vi "GetOpenDataEvents.vi"(8 "error in (no error)":errorcluster, 10 "data group":string, 11 "config":T1) -> (0 "error out":errorcluster, 2 "open data event configs":T2[](array[typedef]), 3 "open data events":T8[](array[typedef]))   [LabVIEW 2017, in "McsaDataEventCreator.lvlib"]
uses:
  <vilib>/addons/InsightCM/Devices/Shared/Mcsa/McsaDataEventCreator/McsaDataEventCreator.lvlib
  <vilib>/addons/InsightCM/Devices/Shared/Common/DataEvent/controls/Event.ctl
  <vilib>/addons/InsightCM/MessageBus/Base/controls/DataEvent.ctl
  <vilib>/addons/InsightCM/MessageBus/Base/controls/KeyValuePair.ctl
  <vilib>/addons/InsightCM/Devices/Shared/Common/DataEvent/controls/DataSet.ctl
  <vilib>/addons/InsightCM/MessageBus/Base/controls/DataSetMetadata.ctl
  <vilib>/addons/InsightCM/MessageBus/Base/controls/TrendPoint.ctl
  <vilib>/addons/InsightCM/MessageBus/Base/controls/TrendAlarmUpdate.ctl
  <vilib>/addons/InsightCM/MessageBus/Base/controls/TrendAlarmTransition.ctl
  <vilib>/addons/InsightCM/Devices/Shared/Mcsa/McsaDataEventCreator/controls/DataEventConfig.ctl
  <vilib>/addons/InsightCM/Devices/Shared/Mcsa/McsaDataEventCreator/controls/AcqParams.ctl
  <vilib>/addons/InsightCM/Devices/Shared/Common/DataAccumulator/controls/AccumulationSettings.ctl
  <vilib>/addons/InsightCM/Devices/Shared/Common/DataAccumulator/controls/accumulationType.ctl
  <vilib>/addons/InsightCM/Devices/Shared/Common/DVRBuffer/controls/BufferLocation.ctl
  <vilib>/addons/PointValueMap/controls/PointMap.ctl
  <vilib>/addons/InsightCM/Devices/Shared/Mcsa/McsaDataEventCreator/controls/config.ctl
  <vilib>/addons/PointValueMap/PointValueMap.lvlib
  <vilib>/addons/InsightCM/Devices/Shared/Common/DVRBuffer/DVRBuffer.lvlib
  <vilib>/addons/InsightCM/Devices/Shared/Common/DataAccumulator/DataAccumulator.lvlib
  <vilib>/addons/InsightCM/Devices/Shared/Common/DataEvent/DataEvent.lvlib
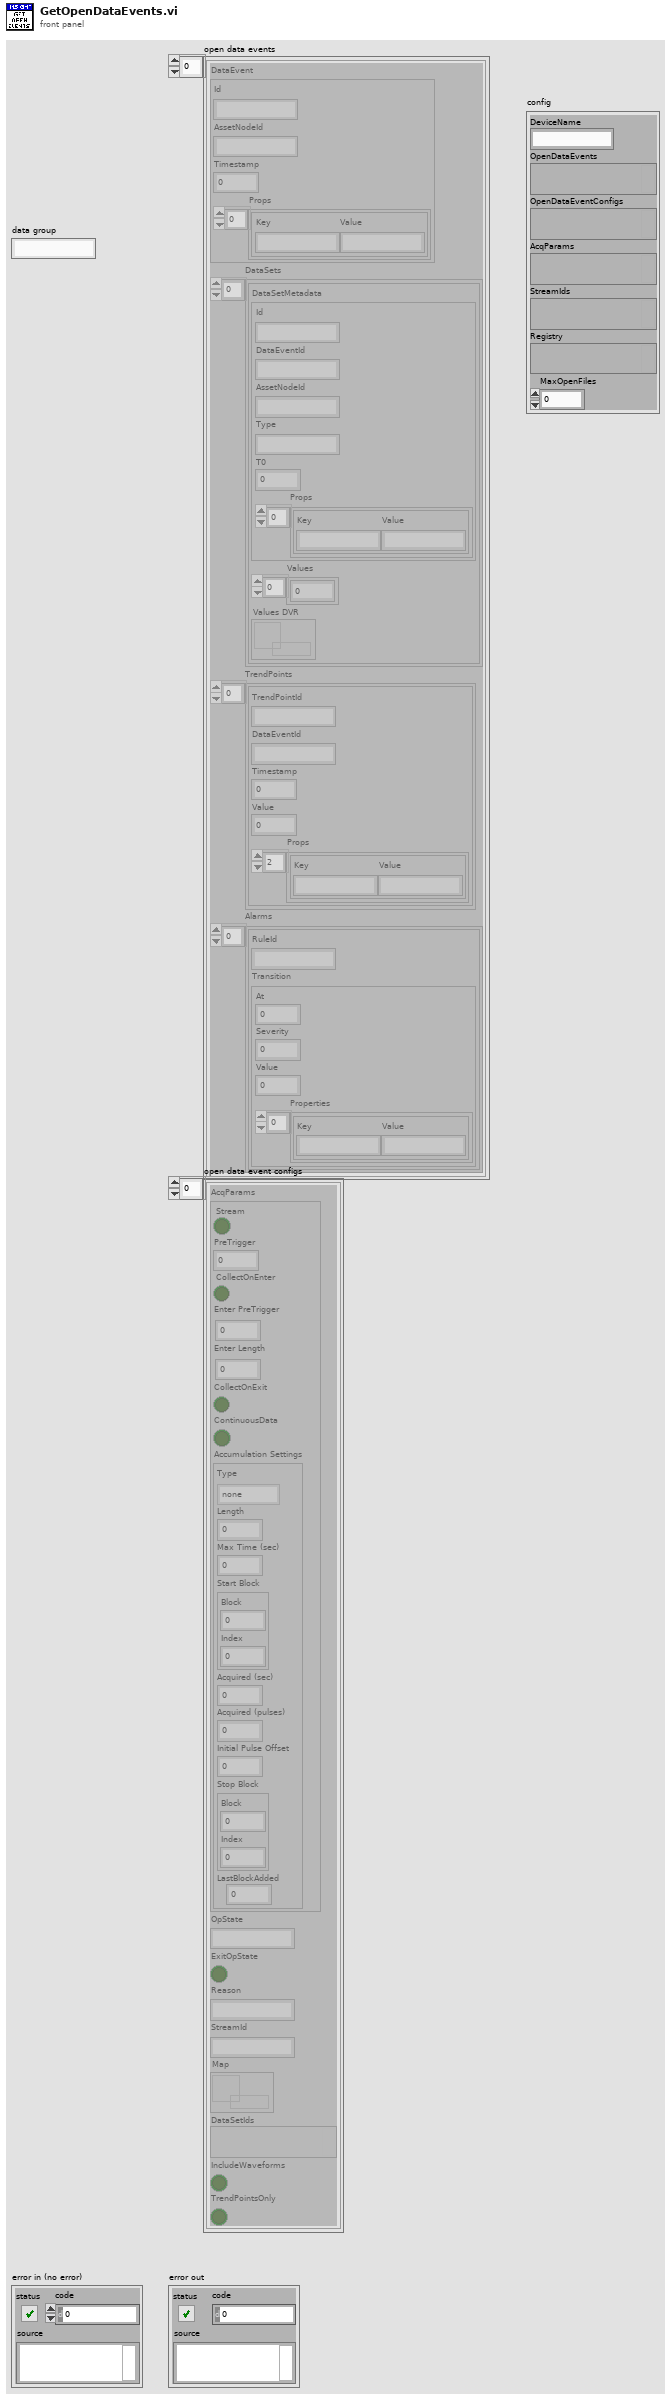
[diagram p1: front panel]
types:
  T1 = typedef "McsaDataEventCreator.lvlib/config.ctl" = cluster{"DeviceName":string, "OpenDataEvents":variant, "OpenDataEventConfigs":variant, "AcqParams":variant, "StreamIds":variant, "Registry":variant, "MaxOpenFiles":i32}
  T2 = typedef "McsaDataEventCreator.lvlib/DataEventConfig.ctl" = cluster{"AcqParams":T3, "OpState":string, "ExitOpState":bool, "Reason":string, "StreamId":string, "Map":T7, "DataSetIds":variant, "IncludeWaveforms":bool, "TrendPointsOnly":bool}
  T3 = typedef "McsaDataEventCreator.lvlib/AcqParams.ctl" = cluster{"Stream":bool, "PreTrigger":i32, "CollectOnEnter":bool, "Enter PreTrigger":i32, "Enter Length":dbl, "CollectOnExit":bool, "ContinuousData":bool, "Accumulation Settings":T4}
  T4 = typedef "DataAccumulator.lvlib/AccumulationSettings.ctl" = cluster{"Type":T5, "Length":dbl, "Max Time (sec)":dbl, "Start Block":T6, "Acquired (sec)":dbl, "Acquired (pulses)":i32, "Initial Pulse Offset":dbl, "Stop Block":T6, "LastBlockAdded":u32}
  T5 = typedef "DataAccumulator.lvlib/accumulationType.ctl" = enum16{"none", "seconds", "revolutions"}
  T6 = typedef "DVRBuffer.lvlib/BufferLocation.ctl" = cluster{"Block":u32, "Index":i32}
  T7 = typedef "PointValueMap.lvlib/PointMap.ctl" = refnum<data-value>
  T8 = typedef "DataEvent.lvlib/Event.ctl" = cluster{"DataEvent":T9, "DataSets":T11[], "TrendPoints":T13[], "Alarms":T14[]}
  T9 = typedef "DataEvent.ctl" = cluster{"Id":string, "AssetNodeId":string, "Timestamp":i64, "Props":T10[]}
  T10 = typedef "KeyValuePair.ctl" = cluster{"Key":string, "Value":string}
  T11 = typedef "DataEvent.lvlib/DataSet.ctl" = cluster{"DataSetMetadata":T12, "Values":sgl[], "Values DVR":refnum<data-value>}
  T12 = typedef "DataSetMetadata.ctl" = cluster{"Id":string, "DataEventId":string, "AssetNodeId":string, "Type":string, "T0":i64, "Props":T10[]}
  T13 = typedef "TrendPoint.ctl" = cluster{"TrendPointId":string, "DataEventId":string, "Timestamp":i64, "Value":dbl, "Props":T10[]}
  T14 = typedef "TrendAlarmUpdate.ctl" = cluster{"RuleId":string, "Transition":T15}
  T15 = typedef "TrendAlarmTransition.ctl" = cluster{"At":i64, "Severity":i32, "Value":dbl, "Properties":T10[]}
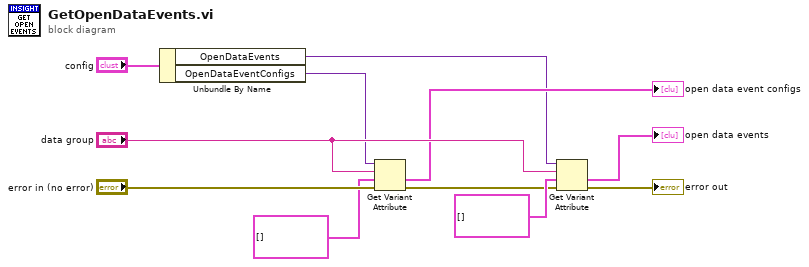
[diagram p0: block diagram]
diagram:
  n1 = Unbundle By Name("config") -> ("OpenDataEvents"=w1:variant, "OpenDataEventConfigs"=w2:variant)
  n2 = Get Variant Attribute(Variant=w2, name="data group", default value (empty Variant)=T2[] [], error in="error in (no error)") -> (value=→"open data event configs":T2[], error out=w7:errorcluster)  [unwired: 2 out]
  n3 = Get Variant Attribute(Variant=w1, name="data group", default value (empty Variant)=T8[] [], error in=w7) -> (value=→"open data events":T8[], error out=→"error out":errorcluster)  [unwired: 2 out]
